vi "MasterStateController.vi"(1 "Selected State":string) -> (0 "Master State":string)   [LabVIEW 2019]
doc: "This is the master robot state controller. The master robot state can affect any of the subsystem state controllers. Inter-system operations such as end-game sequencers should go here."
uses:
  dsdata.vi
  outputs.vi
panel:
  out "State Index":i32
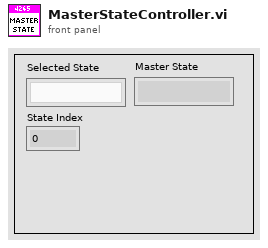
[diagram p1: front panel]
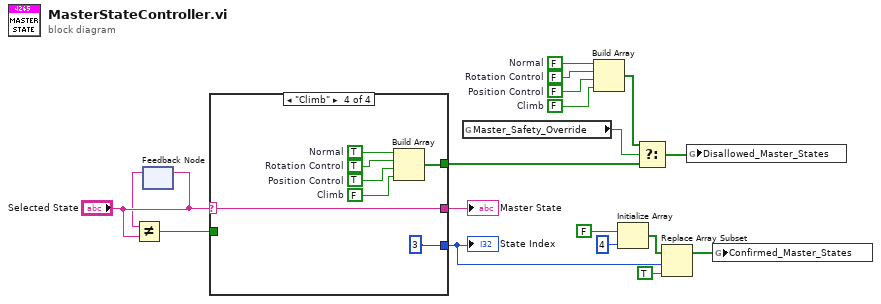
[diagram p0: block diagram]
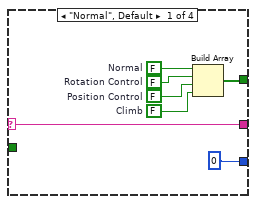
[diagram p2: hidden frame]
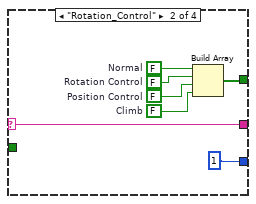
[diagram p3: hidden frame]
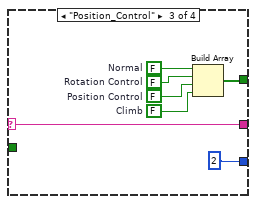
[diagram p4: hidden frame]
diagram:
  w8 = FALSE  # Climb
  w10 = FALSE  # Rotation Control
  w9 = FALSE  # Position Control
  w11 = FALSE  # Normal
  n1 = feedback-in #1("Selected State") -> ()
  n2 = feedback #1() -> (w3:string)  [unwired: 1 in]
  n3 = Not Equal?(x=w3, y="Selected State") -> (x != y?=w2:bool)
  n4 = case shown="\"Climb\"" "Selected State" {
    selector: "Selected State" -> [w24 w31 w38 w45]
    tunnel: [0 ("Index") 1 ("Index") 2 ("Index") 3 ("Index")] -> w15
    tunnel: [w24 w31 w38 w45] -> w12
    tunnel: [w19 w26 w33 w40] -> w5
    tunnel: w2 -> [_ _ _ _]
    frame "Normal", Default {
      w20 = FALSE  # Climb
      w22 = FALSE  # Rotation Control
      w21 = FALSE  # Position Control
      w23 = FALSE  # Normal
      n5 = Build Array(w23, w22, w21, w20) -> (w19:bool[])
    }
    frame "Rotation_Control" {
      w27 = FALSE  # Climb
      w29 = FALSE  # Rotation Control
      w28 = FALSE  # Position Control
      w30 = FALSE  # Normal
      n6 = Build Array(w30, w29, w28, w27) -> (w26:bool[])
    }
    frame "Position_Control" {
      w34 = FALSE  # Climb
      w36 = FALSE  # Rotation Control
      w35 = FALSE  # Position Control
      w37 = FALSE  # Normal
      n7 = Build Array(w37, w36, w35, w34) -> (w33:bool[])
    }
    frame "Climb" {
      w41 = FALSE  # Climb
      w43 = TRUE  # Rotation Control
      w42 = TRUE  # Position Control
      w44 = TRUE  # Normal
      n8 = Build Array(w44, w43, w42, w41) -> (w40:bool[])
    }
  }
  "State Index" <- w15
  "Master State" <- w12
  n9 = global read "dsdata.vi" "Master_Safety_Override"() -> (w7:bool)
  n10 = Build Array(w11, w10, w9, w8) -> (w6:bool[])
  n11 = Initialize Array(FALSE, 4 ("dimension size")) -> (w16:bool[])
  n12 = Select(t=w6, s=w7, f=w5) -> (s? t:f=w1:bool[])
  n13 = Replace Array Subset(array=w16, new element=TRUE ("new element/subarray"), index=w15) -> (w13:bool[])
  n14 = global write "outputs.vi" "Disallowed_Master_States"(w1) -> ()
  n15 = global write "outputs.vi" "Confirmed_Master_States"(w13) -> ()
